vi "read_size.vi"(11 "Bytes in":refnum<class "Bytes.lvclass">) -> (2 "length":i32, 3 "Bytes out":refnum<class "Bytes.lvclass">)   [LabVIEW 2020, in "lvdata.lvlib" / "Bytes.lvclass"]
uses:
  Bytes.lvclass
  Bytes.lvclass/Bytes.ctl
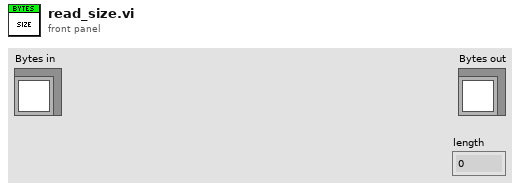
[diagram p1: front panel]
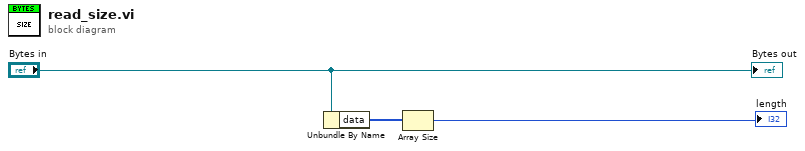
[diagram p0: block diagram]
diagram:
  n1 = Unbundle By Name("Bytes in") -> ("data"=w1:u8[])
  n2 = Array Size(array=w1) -> (size(s)=→"length":i32)
  "Bytes out" <- "Bytes in"
